vi "Blind Navigation Glove Final.vi"() -> ()   [LabVIEW 2022 SP3]
uses:
  <vilib>/MakerHub/LINX/Private/Device/Type Defs/Stimulus Pulse.ctl
  <vilib>/DAQmx/read.llb/DAQmx Read (Analog 1D DBL NChan 1Samp).vi
  <vilib>/DAQmx/write.llb/DAQmx Write (Digital Bool 1Line 1Point).vi
  <vilib>/DAQmx/create/channels.llb/DAQmx Create Channel (DO-Digital Output).vi
  <vilib>/DAQmx/miscellaneous.llb/DAQmx Fill In Error Info.vi
  <vilib>/MakerHub/LINX/Public/Utilities/Open Serial.vi
  <vilib>/DAQmx/create/channels.llb/DAQmx Create Channel (AI-Voltage-Basic).vi
  <vilib>/MakerHub/LINX/LMH-LINX.lvlib
  <vilib>/httpClient/LabVIEWHTTPClient.lvlib
  <vilib>/MakerHub/LINX/Private/Device/Device.lvlib
panel:
  out "Vibrator":bool
  out "Average Distance(cm)":dbl
  in  "stop 4":bool
  out "String":string
  in  "Vibrator Output":tag
  in  "Echo":u8
  out "Pulse Width (uS)":u32
  out "Distance(cm)":dbl
  in  "stop 3":bool
  in  "Serial Port":refnum<visa-resource-name>="N/A"
  in  "Trig":u8
  out "Buzzer":bool
  out "Average Temperature(°C)":dbl(knob) scale=0.0..45.0
  out "LM35 Ouptput":dbl
  out "Current Temperature(°C)":dbl(knob) scale=0.0..45.0
  in  "stop 2":bool
  in  "Buzzer Ouput":tag
  in  "stop":bool
  out "Voltage Output 2":dbl
  out "Voltage Output 1":dbl
  out "Elapsed Time 2":dbl
  in  "Timer 2":bool
  out "Digital Control 2":bool
  out "Control Signal 2":bool
  out "2. Voltage less than 1?":bool
  out "Input Voltage 2":dbl(knob) scale=-5.0..5.0
  out "Elapsed Time":dbl
  out "Control Signal 1":bool
  out "Digital Control 1":bool
  out "Voltage less than 1?":bool
  in  "Timer 1":bool
  in  "Main Loop":bool
  out "Input Voltage 1":dbl(knob) scale=-5.0..5.0
  in  "Analog Input channel":tag
  # "Tempereature Sensor"
  # "Flex Sensor 01"
  # "Flex Sensor 02"
  # "Ultrasonic Sensor"
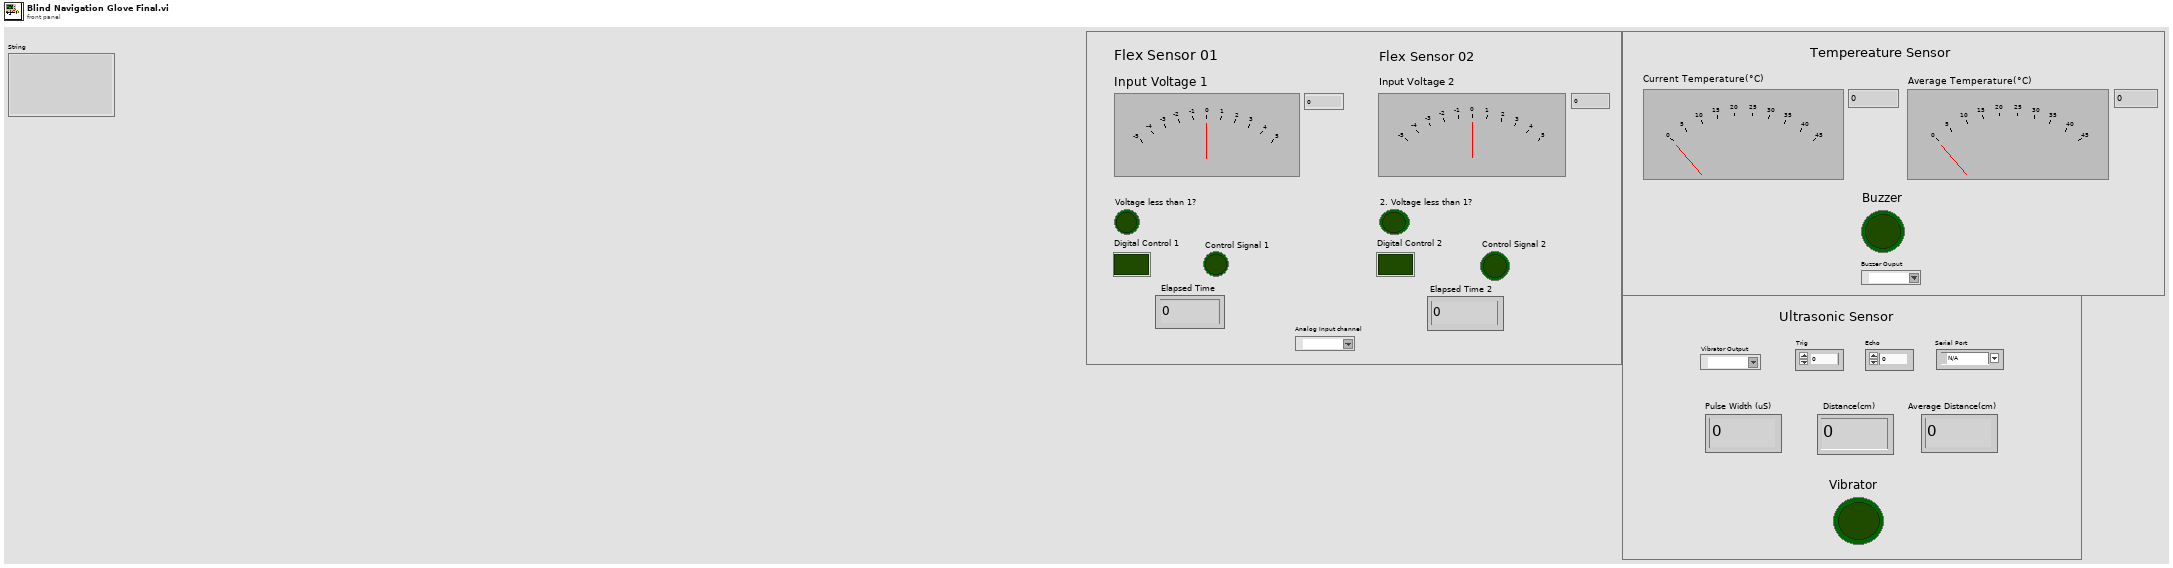
[diagram p1: front panel]
types:
  T1 = typedef "LMH-LINX.lvlib/LINX Ref.ctl" = cluster{"IO":T2, "Interface":T3, "LINX Device Config":T4}
  T2 = typedef "LMH-LINX.lvlib/Platform.ctl" = enum16{"Remote", "Local"}
  T3 = typedef "LMH-LINX.lvlib/Interface.ctl" = enum16{"Serial", "TCP"}
  T4 = typedef "LMH-LINX.lvlib/Device.lvlib/LINX Device Config.ctl" = cluster{"Interface":T3, "COM Port":refnum<visa-resource-name>, "TCP Configuration":T5, "Device Family":u8, "Device ID":u8, "Device Name":string, "TCP Ref":refnum<k5>, "Channels":T6}
  T5 = typedef "LMH-LINX.lvlib/Device.lvlib/TCP Config.ctl" = cluster{"IP Address":string, "Port":u16}
  T6 = typedef "LMH-LINX.lvlib/Channels.ctl" = cluster{"DI":u8[], "DO":u8[], "AI":u8[], "AO":u8[], "PWM":u8[], "QE":u8[], "UART":u8[], "I2C 2":u8[], "SPI":u8[], "CAN":u8[], "Servo":u8[], "AI Ref (V)":dbl, "AI Resolution (Bits)":u8, "AO Ref (V)":dbl, "AO Resolution (Bits)":u8}
  T7 = typedef "LMH-LINX.lvlib/Device.lvlib/Stimulus Pulse.ctl" = enum16{"None", "Active Low", "Active High"}
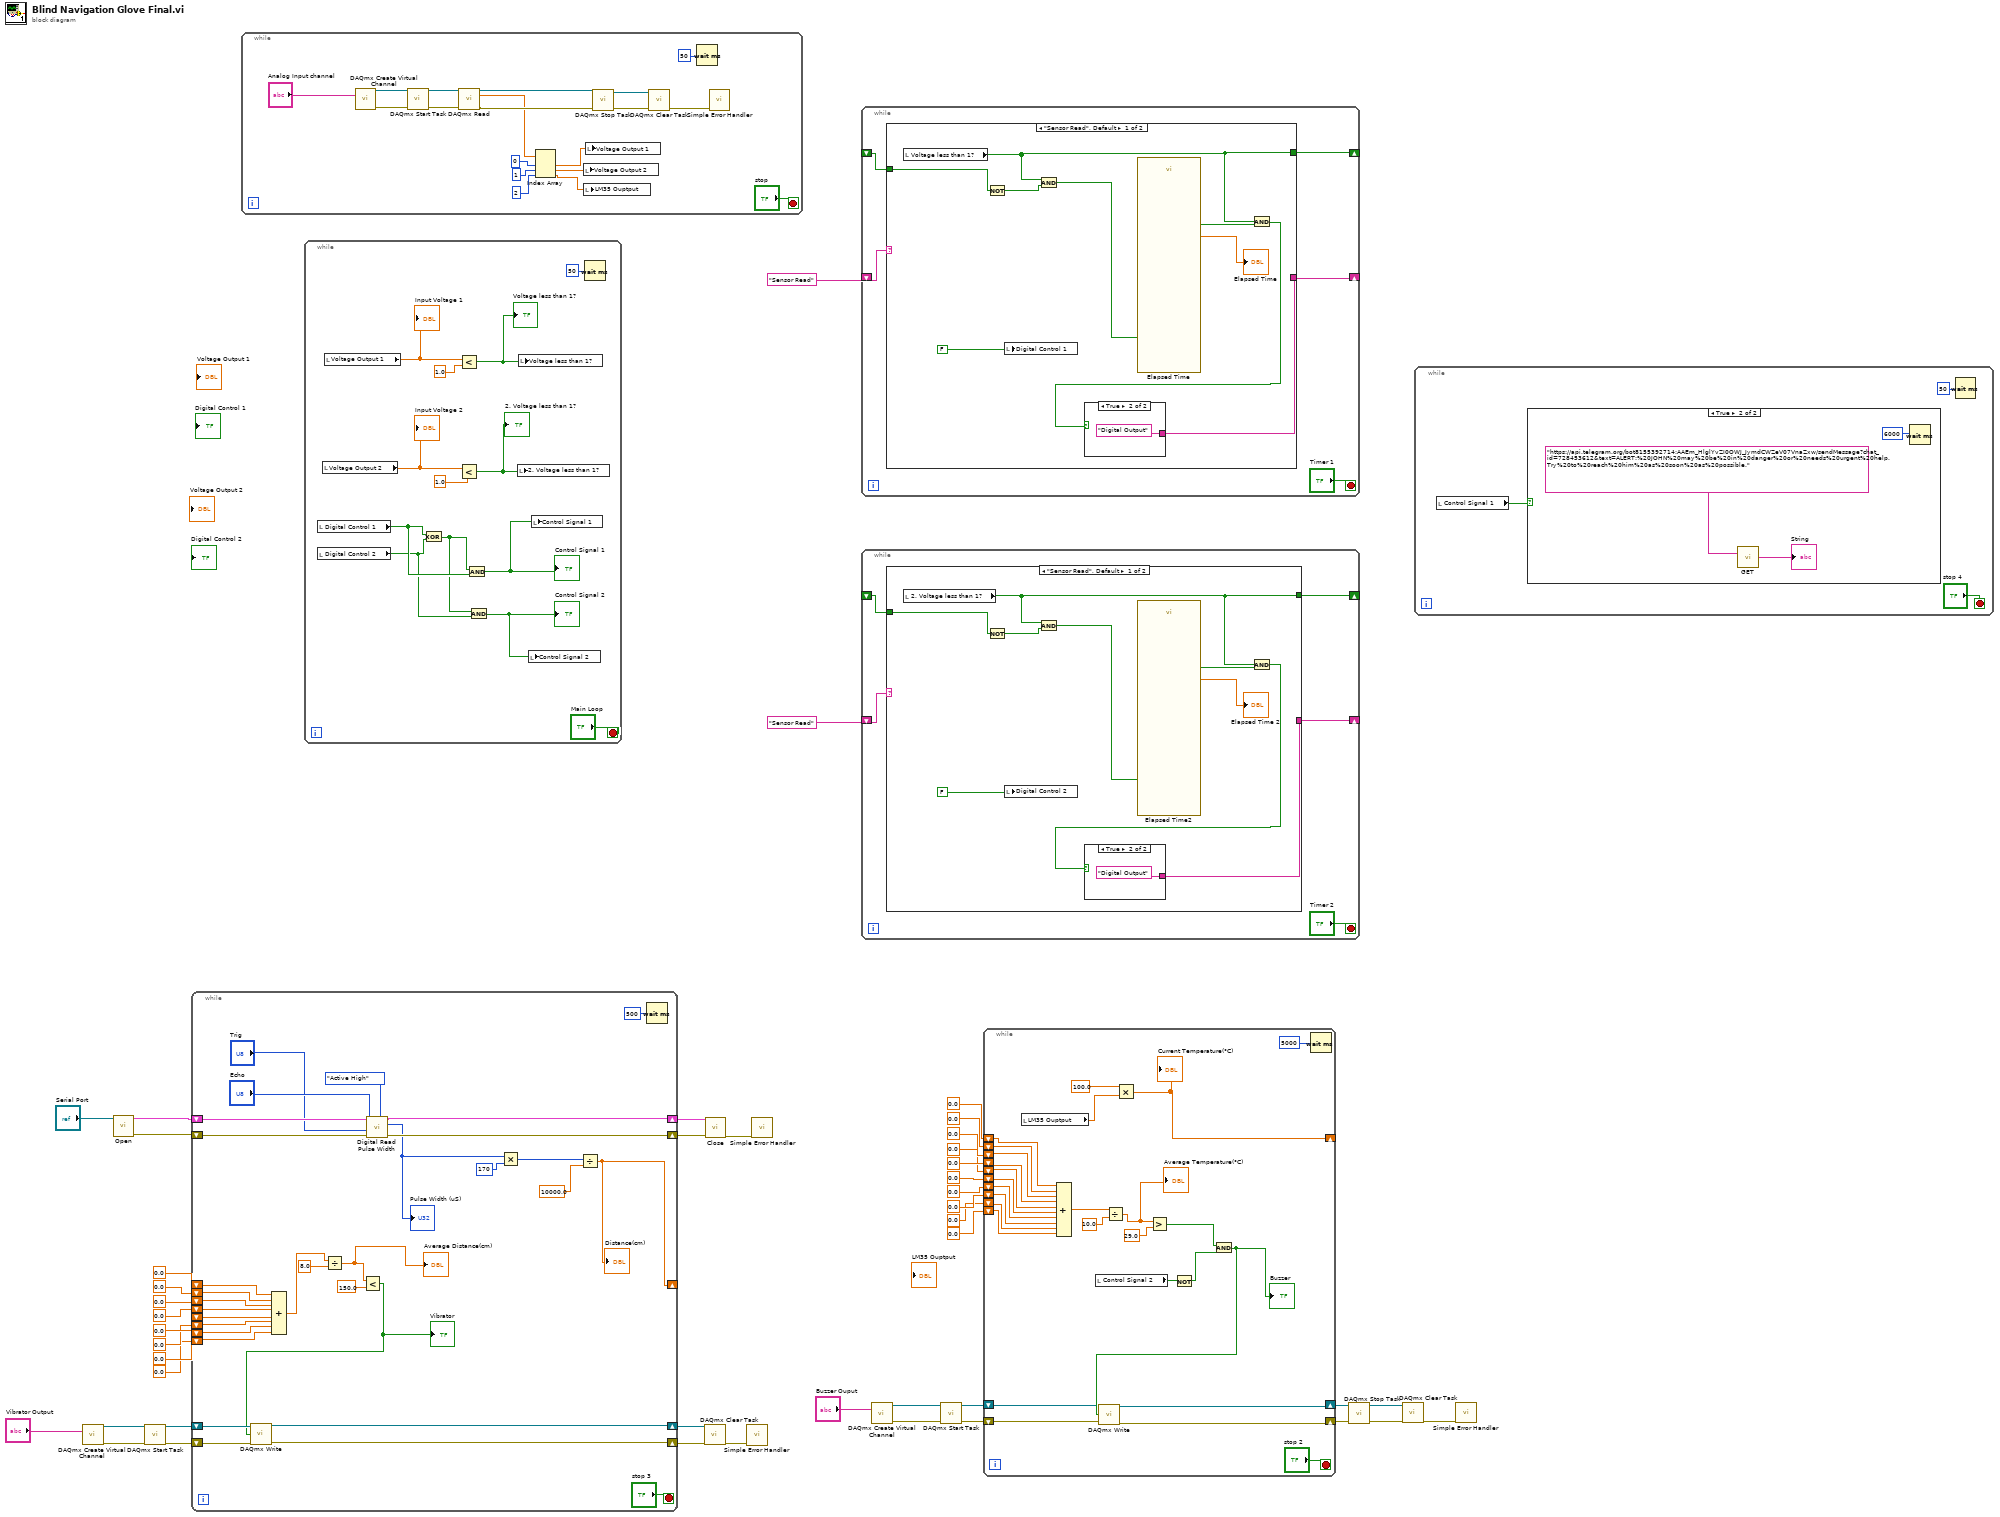
[diagram p0: block diagram]
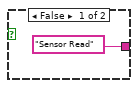
[diagram p3: hidden frame]
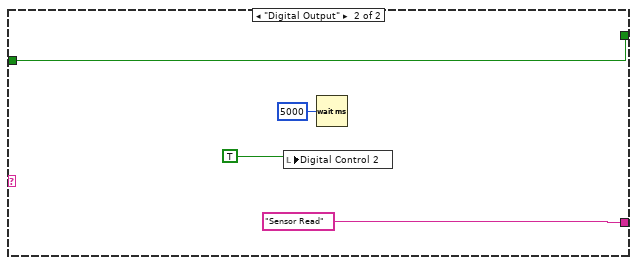
[diagram p4: hidden frame]
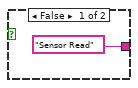
[diagram p5: hidden frame]
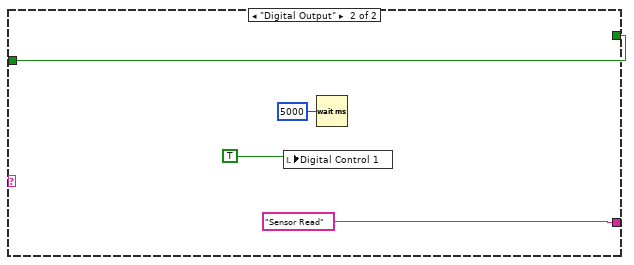
[diagram p6: hidden frame]
diagram:
  n1 = call-poly <vilib>:"DAQmx Create Virtual Channel.vi"("lines"="Vibrator Output") -> ("task out"=w10:refnum<k21>, "error out"=w9:errorcluster)  [unwired: 13 in]
  n2 = call-poly <vilib>:"Open.vi"("Serial Port"="Serial Port") -> ("Error Out"=w1:errorcluster, "LINX Resource"=w21:T1)  [unwired: 8 in, 1 out]
  n3 = call <vilib>:"DAQmx Start Task.vi"("task/channels in"=w10, "error in"=w9) -> ("task out"=w8:refnum<k21>, "error out"=w7:errorcluster)  [unwired: 12 in]
  n4 = while {
    shift-right: [w56] -> _
    shift-left: 0.0 -> [w55]
    shift-left: 0.0 -> [w54]
    shift-left: 0.0 -> [w53]
    shift-left: 0.0 -> [w52]
    shift-left: 0.0 -> [w51]
    shift-left: 0.0 -> [w50]
    shift-left: 0.0 -> [w49]
    shift-left: 0.0 -> [w48]
    shift-right: [w59] -> w3
    shift-left: w21 -> [w70]
    shift-right: [w58] -> w2
    shift-left: w1 -> [w69]
    shift-right: [w62] -> w6
    shift-left: w8 -> [w64]
    shift-right: [w61] -> w5
    shift-left: w7 -> [w63]
    stop <- "stop 3" stop-if-true
    n5 = Compound Arithmetic op=ADD(w55, w54, w53, w52, w51, w50, w49, w48) -> (w67:dbl)
    n6 = Divide(x=w67, y=8.0) -> (x/y=w46:dbl)
    "Average Distance(cm)" <- w46
    n7 = Less?(x=w46, y=150.0) -> (x < y?=w45:bool)
    "Vibrator" <- w45
    n8 = call-poly <vilib>:"DAQmx Write.vi"("task/channels in"=w64, "data"=w45, "error in"=w63) -> ("task out"=w62:refnum<k21>, "error out"=w61:errorcluster)  [unwired: 10 in, 1 out]
    n9 = call <vilib>:"Digital Read Pulse Width.vi"("Stimulus Pulse (Active High)"=Stimulus_Pulse."Active High", "Error In"=w69, "DO Channel"="Trig", "DI Channel"="Echo", "LINX Resource"=w70) -> ("Error Out"=w58:errorcluster, "Pulse Width (uS)"=w57:u32, "LINX Resource"=w59:T1)  [unwired: 4 in]
    "Pulse Width (uS)" <- w57
    n10 = Multiply(x=w57, y=u32 170) -> (x*y=w71:u32)
    n11 = Divide(x=w71, y=10000.0) -> (x/y=w56:dbl)
    "Distance(cm)" <- w56
    n12 = Wait (ms)(milliseconds to wait=u32 500) -> ()  [unwired: 1 out]
  }
  n13 = while {
    stop <- "stop" stop-if-true
    n14 = call-poly <vilib>:"DAQmx Create Virtual Channel.vi"("physical channels"="Analog Input channel") -> ("task out"=w84:refnum<k21>, "error out"=w85:errorcluster)  [unwired: 13 in]
    n15 = call <vilib>:"DAQmx Start Task.vi"("task/channels in"=w84, "error in"=w85) -> ("task out"=w86:refnum<k21>, "error out"=w87:errorcluster)  [unwired: 12 in]
    n16 = call-poly <vilib>:"DAQmx Read.vi"("task/channels in"=w86, "error in"=w87) -> ("task out"=w78:refnum<k21>, "data"=w77:dbl[], "error out"=w93:errorcluster)  [unwired: 11 in]
    n17 = Index Array(array=w77, index #1=0 ("index"), index #2=1 ("index"), index #3=2 ("index")) -> (element #1=w91:dbl, element #2=w92:dbl, element #3=w76:dbl)
    n18 = local write "Voltage Output 2"(w92) -> ()
    n19 = local write "LM35 Ouptput"(w76) -> ()
    n20 = local write "Voltage Output 1"(w91) -> ()
    n21 = call <vilib>:"DAQmx Stop Task.vi"("task/channels in"=w78, "error in"=w93) -> ("task out"=w88:refnum<k21>, "error out"=w89:errorcluster)  [unwired: 12 in]
    n22 = call <vilib>:"DAQmx Clear Task.vi"("task in"=w88, "error in"=w89) -> ("error out"=w90:errorcluster)  [unwired: 13 in]
    n23 = Wait (ms)(milliseconds to wait=u32 50) -> ()  [unwired: 1 out]
    n24 = call <vilib>:"Simple Error Handler.vi"("error in (no error)"=w90) -> ()  [unwired: 4 in, 5 out]
  }
  n25 = while {
    stop <- "Main Loop" stop-if-true
    n26 = local read "Digital Control 1"() -> (w101:bool)
    n27 = local read "Digital Control 2"() -> (w99:bool)
    n28 = local read "Voltage Output 2"() -> (w103:dbl)
    "Input Voltage 2" <- w103
    n29 = local read "Voltage Output 1"() -> (w102:dbl)
    "Input Voltage 1" <- w102
    n30 = Exclusive Or(1:w99, 2:w101) -> (0:w100:bool)
    n31 = Less?(x=w102, y=1.0) -> (x < y?=w96:bool)
    "Voltage less than 1?" <- w96
    n32 = Less?(x=w103, y=1.0) -> (x < y?=w95:bool)
    "2. Voltage less than 1?" <- w95
    n33 = And(x=w100, y=w101) -> (x .and. y?=w97:bool)
    "Control Signal 1" <- w97
    n34 = And(x=w100, y=w99) -> (x .and. y?=w98:bool)
    "Control Signal 2" <- w98
    n35 = local write "2. Voltage less than 1?"(w95) -> ()
    n36 = local write "Voltage less than 1?"(w96) -> ()
    n37 = local write "Control Signal 2"(w98) -> ()
    n38 = local write "Control Signal 1"(w97) -> ()
    n39 = Wait (ms)(milliseconds to wait=u32 50) -> ()  [unwired: 1 out]
  }
  n40 = call <vilib>:"DAQmx Clear Task.vi"("task in"=w6, "error in"=w5) -> ("error out"=w4:errorcluster)  [unwired: 13 in]
  n41 = call <vilib>:"Close.vi"("Error In"=w2, "LINX Resource"=w3) -> ("Error Out"=w20:errorcluster)  [unwired: 9 in]
  n42 = call <vilib>:"Simple Error Handler.vi"("error in (no error)"=w4) -> ()  [unwired: 4 in, 5 out]
  n43 = call <vilib>:"Simple Error Handler.vi"("error in (no error)"=w20) -> ()  [unwired: 4 in, 5 out]
  n44 = while {
    shift-right: [w111] -> _
    shift-left: "Sensor Read" -> [w112]
    shift-right: [w108] -> _
    shift-left: _ -> [w109]
    stop <- "Timer 1" stop-if-true
    n45 = case shown="\"Sensor Read\", Default" w112 {
      tunnel: [w121 "Sensor Read"] -> w111
      tunnel: [w113 w125] -> w108
      tunnel: w109 -> [w116 w125]
      frame "Sensor Read", Default {
        n46 = local read "Voltage less than 1?"() -> (w113:bool)
        n47 = Not(x=w116) -> (.not. x?=w115:bool)
        n48 = local write "Digital Control 1"(FALSE) -> ()
        n49 = And(x=w113, y=w115) -> (x .and. y?=w120:bool)
        n50 = call "Elapsed Time"("Reset"=w120) -> ("Elapsed Time (s)"=→"Elapsed Time":dbl, "Time has Elapsed"=w119:bool)  [unwired: 11 in, 6 out]
        n51 = And(x=w113, y=w119) -> (x .and. y?=w118:bool)
        n52 = case shown="True" w118 {
          tunnel: ["Sensor Read" "Digital Output"] -> w121
          frame False {
          }
          frame True {
          }
        }
      }
      frame "Digital Output" {
        n53 = local write "Digital Control 1"(TRUE) -> ()
        n54 = Wait (ms)(milliseconds to wait=u32 5000) -> ()  [unwired: 1 out]
      }
    }
  }
  n55 = while {
    shift-right: [w131] -> _
    shift-left: "Sensor Read" -> [w132]
    shift-right: [w128] -> _
    shift-left: _ -> [w129]
    stop <- "Timer 2" stop-if-true
    n56 = case shown="\"Sensor Read\", Default" w132 {
      tunnel: [w141 "Sensor Read"] -> w131
      tunnel: [w133 w145] -> w128
      tunnel: w129 -> [w136 w145]
      frame "Sensor Read", Default {
        n57 = local read "2. Voltage less than 1?"() -> (w133:bool)
        n58 = Not(x=w136) -> (.not. x?=w135:bool)
        n59 = local write "Digital Control 2"(FALSE) -> ()
        n60 = And(x=w133, y=w135) -> (x .and. y?=w140:bool)
        n61 = call "Elapsed Time2"("Reset"=w140) -> ("Elapsed Time (s)"=→"Elapsed Time 2":dbl, "Time has Elapsed"=w139:bool)  [unwired: 11 in, 6 out]
        n62 = And(x=w133, y=w139) -> (x .and. y?=w138:bool)
        n63 = case shown="True" w138 {
          tunnel: ["Sensor Read" "Digital Output"] -> w141
          frame False {
          }
          frame True {
          }
        }
      }
      frame "Digital Output" {
        n64 = local write "Digital Control 2"(TRUE) -> ()
        n65 = Wait (ms)(milliseconds to wait=u32 5000) -> ()  [unwired: 1 out]
      }
    }
  }
  n66 = call-poly <vilib>:"DAQmx Create Virtual Channel.vi"("lines"="Buzzer Ouput") -> ("task out"=w38:refnum<k21>, "error out"=w37:errorcluster)  [unwired: 13 in]
  n67 = call <vilib>:"DAQmx Start Task.vi"("task/channels in"=w38, "error in"=w37) -> ("task out"=w36:refnum<k21>, "error out"=w35:errorcluster)  [unwired: 12 in]
  n68 = while {
    shift-right: [w149] -> w34
    shift-left: w36 -> [w151]
    shift-right: [w150] -> w33
    shift-left: w35 -> [w152]
    shift-right: [w172] -> _
    shift-left: 0.0 -> [w171]
    shift-left: 0.0 -> [w170]
    shift-left: 0.0 -> [w169]
    shift-left: 0.0 -> [w168]
    shift-left: 0.0 -> [w167]
    shift-left: 0.0 -> [w166]
    shift-left: 0.0 -> [w165]
    shift-left: 0.0 -> [w164]
    shift-left: 0.0 -> [w163]
    shift-left: 0.0 -> [w162]
    stop <- "stop 2" stop-if-true
    n69 = local read "LM35 Ouptput"() -> (w173:dbl)
    n70 = Compound Arithmetic op=ADD(w171, w170, w169, w168, w167, w166, w165, w164, w163, w162) -> (w161:dbl)
    n71 = local read "Control Signal 2"() -> (w155:bool)
    n72 = Divide(x=w161, y=10.0) -> (x/y=w158:dbl)
    "Average Temperature(°C)" <- w158
    n73 = Multiply(x=100.0, y=w173) -> (x*y=w172:dbl)
    "Current Temperature(°C)" <- w172
    n74 = Greater?(x=w158, y=29.0) -> (0:w156:bool)
    n75 = Not(x=w155) -> (.not. x?=w154:bool)
    n76 = And(x=w156, y=w154) -> (x .and. y?=w153:bool)
    "Buzzer" <- w153
    n77 = call-poly <vilib>:"DAQmx Write.vi"("task/channels in"=w151, "data"=w153, "error in"=w152) -> ("task out"=w149:refnum<k21>, "error out"=w150:errorcluster)  [unwired: 10 in, 1 out]
    n78 = Wait (ms)(milliseconds to wait=u32 5000 ("millisecond timer value")) -> ()  [unwired: 1 out]
  }
  n79 = call <vilib>:"DAQmx Stop Task.vi"("task/channels in"=w34, "error in"=w33) -> ("task out"=w41:refnum<k21>, "error out"=w39:errorcluster)  [unwired: 12 in]
  n80 = call <vilib>:"DAQmx Clear Task.vi"("task in"=w41, "error in"=w39) -> ("error out"=w40:errorcluster)  [unwired: 13 in]
  n81 = while {
    stop <- "stop 4" stop-if-true
    n82 = local read "Control Signal 1"() -> (w175:bool)
    n83 = case shown="True" w175 {
      frame False {
      }
      frame True {
        n84 = call <vilib>:"GET.vi"("url"="https://api.telegram.org/bot8155392714:AAEm_HlglYvZI0OWJ_JymdCWZeV07VnaZxw/sendMessage?chat_id=728453612&text=ALERT:%20JOHN%20may%20be%20in%20danger%20or%20needs%20urgent%20help.Try%20to%20reach%20him%20as%20soon%20as%20possible.") -> ("body"=→"String":string)  [unwired: 11 in, 3 out]
        n85 = Wait (ms)(milliseconds to wait=u32 6000 ("millisecond timer value")) -> ()  [unwired: 1 out]
      }
    }
    n86 = Wait (ms)(milliseconds to wait=u32 50) -> ()  [unwired: 1 out]
  }
  n87 = call <vilib>:"Simple Error Handler.vi"("error in (no error)"=w40) -> ()  [unwired: 4 in, 5 out]
